vi "Config.vi"(8 "error in (no error)":errorcluster, 9 "Read only?":bool, 11 "STEP in":T1) -> (0 "error out":errorcluster, 1 "Discard?":bool=TRUE, 3 "STEP out":T1)   [LabVIEW 2014, in "SeqLoop.lvlib"]
uses:
  SeqLoop.lvlib
  TypeDefs/STEP.ctl
  TypeDefs/LogicParsedExpression.ctl
  Mimico Display/TypeDefs/Mimic Data.ctl
  Mimico Display/TypeDefs/BG Image.ctl
  Mimico Display/TypeDefs/mObject.ctl
  <vilib>/Utility/miscctls.llb/LVPointTypeDef.ctl
  Mimico Display/Mimico Display.lvlib
panel:
  in  "Reset?":bool
  in  "Number of STEPs":u32 caption="Cantidad de Pasos:"
  in  "Jump?":bool caption="Salto de Paso?"
  in  "Repetition":u32 caption="Nro. Repeticiones:"
  in  "Initial STEP":u32 caption="Punto de Salto:"
  out "Mimic Picture":picture
  in  "Mensaje de Error":string
  in  "Add Mimic":bool
  in  "Alarm Msj 4":string
  in  "Alarm Msj 3":string
  in  "Alarm Msj 2":string
  in  "Alarm Msj 1":string
  in  "Alarm 4":string
  in  "Alarm 3":string
  in  "Alarm 2":string
  in  "Alarm 1":string
  out "Paso:":u32
  in  "Mensaje al Operador":string
  in  "Condición de Error":string
  in  "S8:":i32
  in  "S7:":i32
  in  "S6:":i32
  in  "S5:":i32
  in  "S4:":i32
  in  "S3:":i32
  in  "S2:":i32
  in  "S1:":i32
  in  "Condición de Avance de Secuencia":string
  in  "Stop Med":bool
  in  "Add Med":bool
  # "Salto de Paso o Reset"
  # "Salidas Activadas"
  # "Gráfico Mimico"
  # "Alarma"
  # "Mensaje de Alarma"
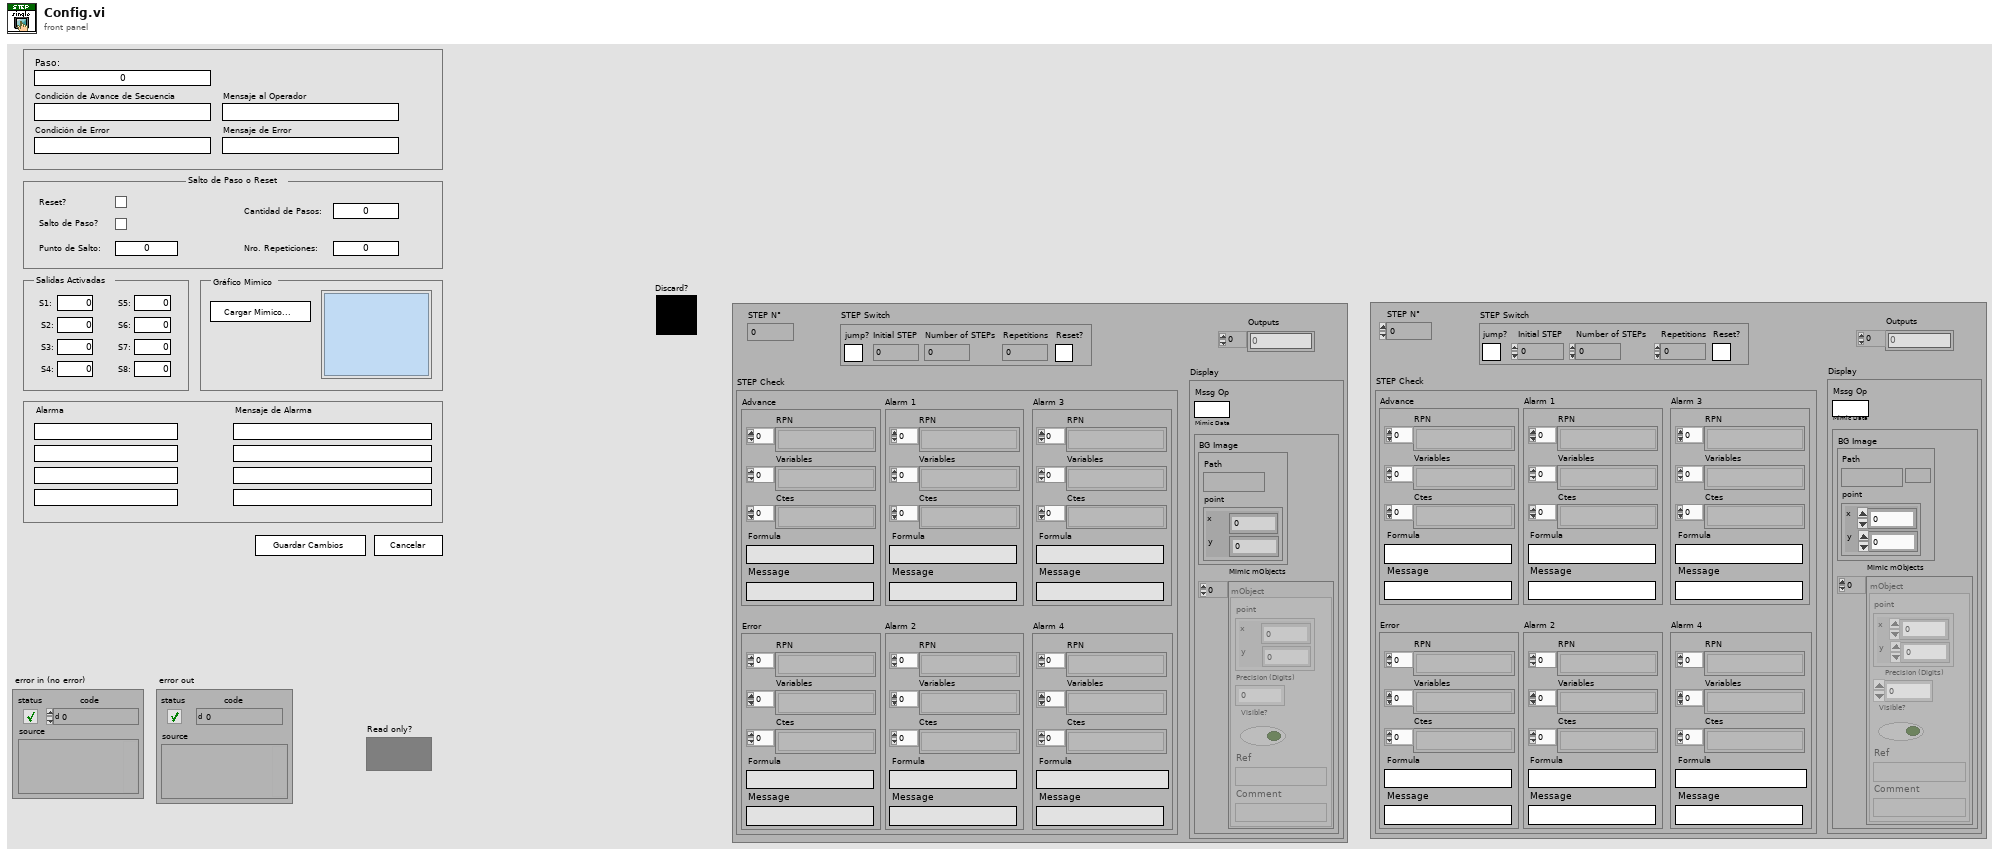
[diagram p1: front panel]
types:
  T1 = typedef "SeqLoop.lvlib/STEP.ctl" = cluster{"STEP N°":u32, "STEP Switch":cluster{"jump?":bool, "Initial STEP":u32, "Number of STEPs":u32, "Repetitions":u32, "Reset?":bool}, "Outputs":i32[], "STEP Check":cluster{"Advance":T2, "Error ":T2, "Alarm 1":T2, "Alarm 2":T2, "Alarm 3":T2, "Alarm 4":T2}, "Display":cluster{"Mssg Op":string, "Mimic Data":T3}}
  T2 = typedef "SeqLoop.lvlib/LogicParsedExpression.ctl" = cluster{"RPN ":string[], "Variables":string[], "Ctes":string[], "Formula":string, "Message":string}
  T3 = typedef "SeqLoop.lvlib/Mimico Display.lvlib/Mimic Data.ctl" = cluster{"BG Image":T4, "Mimic mObjects":T5[]}
  T4 = typedef "SeqLoop.lvlib/Mimico Display.lvlib/BG Image.ctl" = cluster{"Path":path, "point":cluster{"x":i16, "y":i16}}
  T5 = typedef "SeqLoop.lvlib/Mimico Display.lvlib/mObject.ctl" = cluster{"point":cluster{"x":i16, "y":i16}, "Precision (Digits)":i32, "Visible?":bool, "Ref":string, "Comment":string}
  T6 = typedef "LVPointTypeDef.ctl" = cluster{"Horizontal":i16, "Vertical":i16}
  T7 = enum8{"Enabled", "Disabled", "Disabled and Grayed Out"}
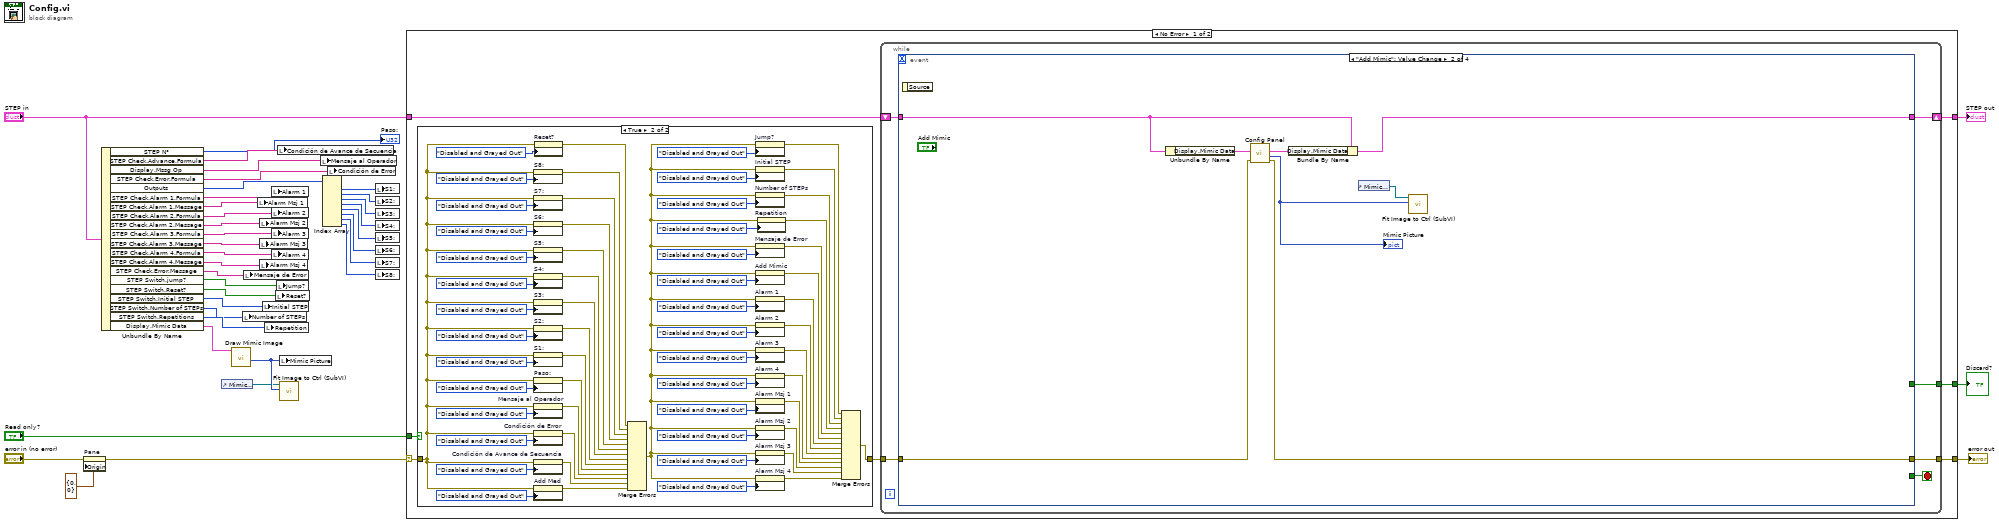
[diagram p0: block diagram]
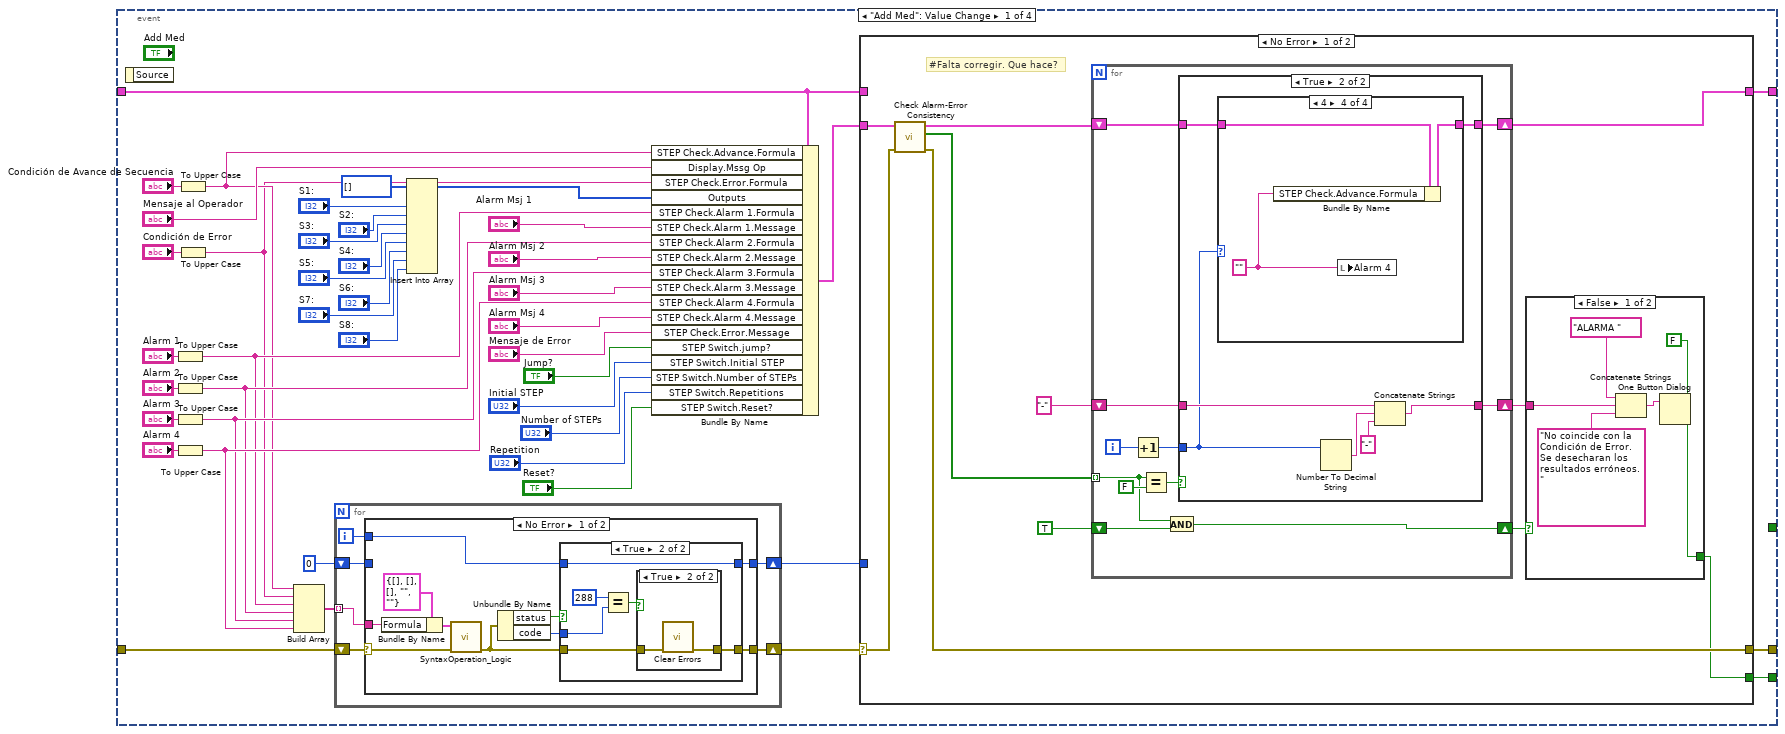
[diagram p3: hidden frame]
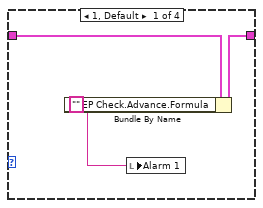
[diagram p5: hidden frame]
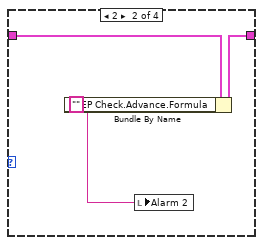
[diagram p6: hidden frame]
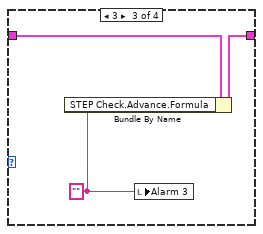
[diagram p7: hidden frame]
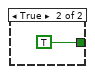
[diagram p8: hidden frame]
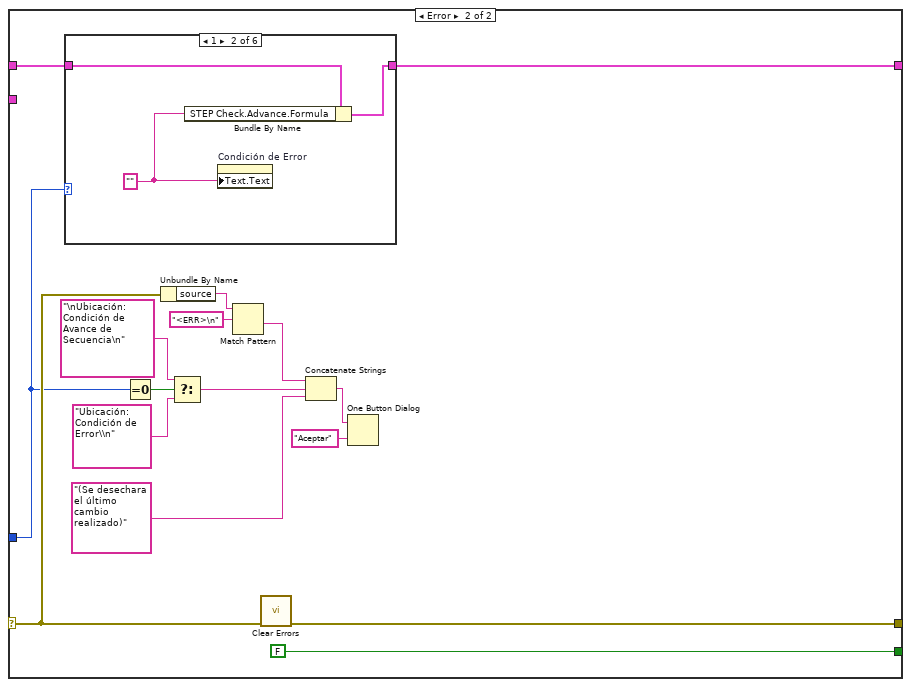
[diagram p9: hidden frame]
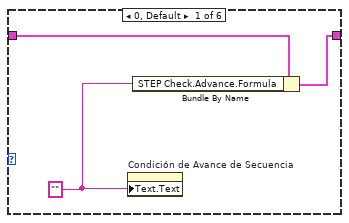
[diagram p10: hidden frame]
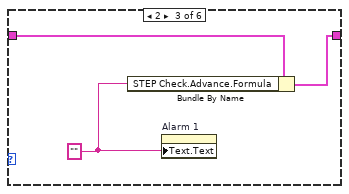
[diagram p11: hidden frame]
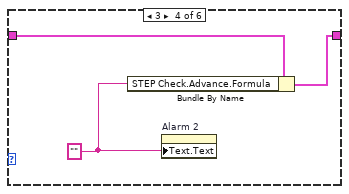
[diagram p12: hidden frame]
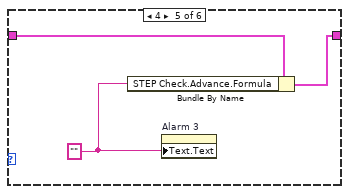
[diagram p13: hidden frame]
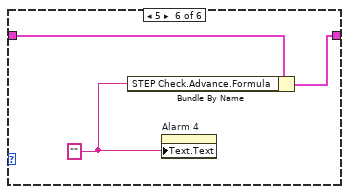
[diagram p14: hidden frame]
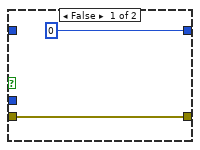
[diagram p15: hidden frame]
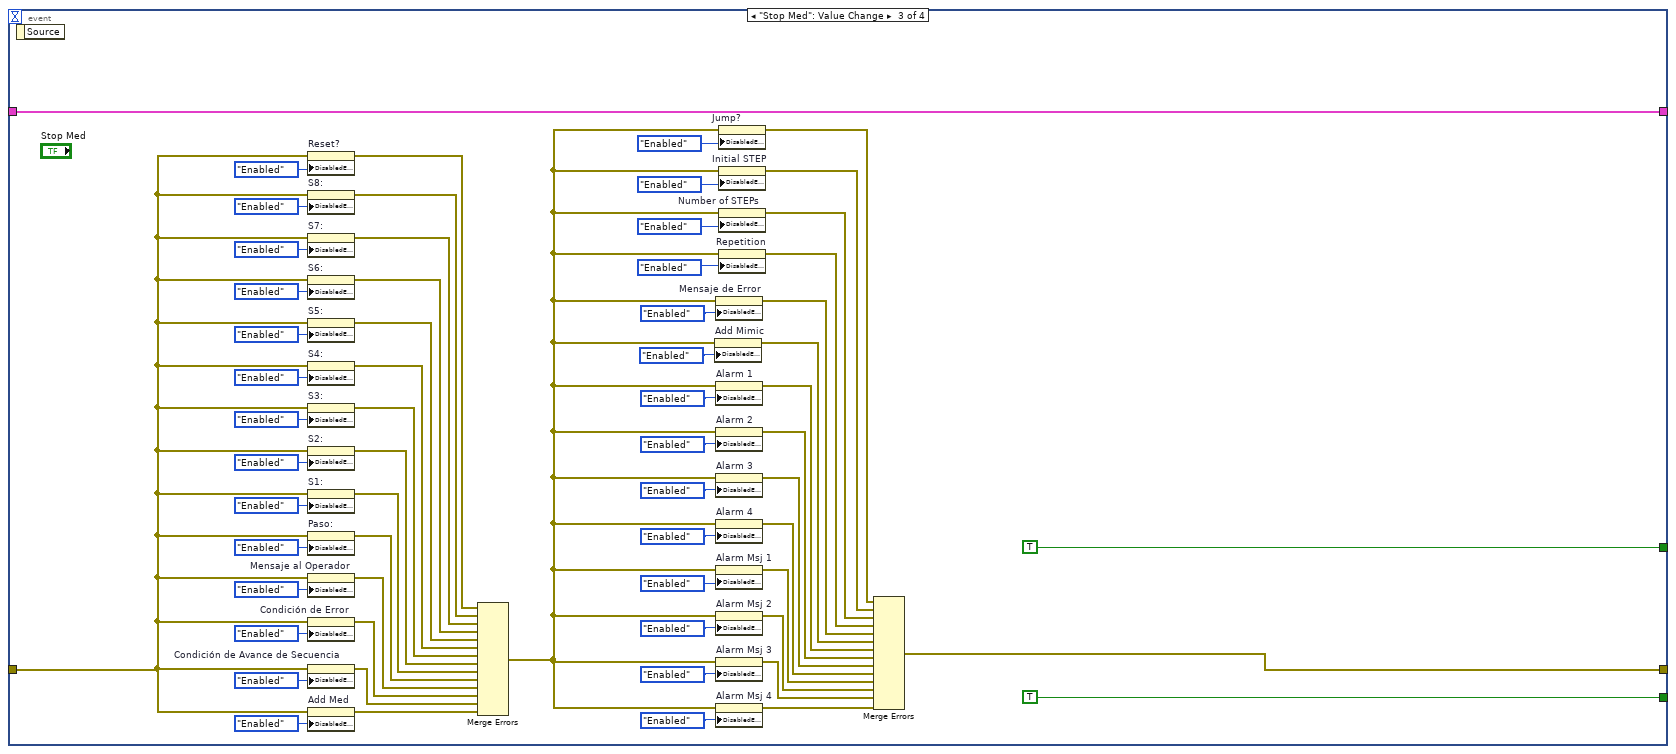
[diagram p18: hidden frame]
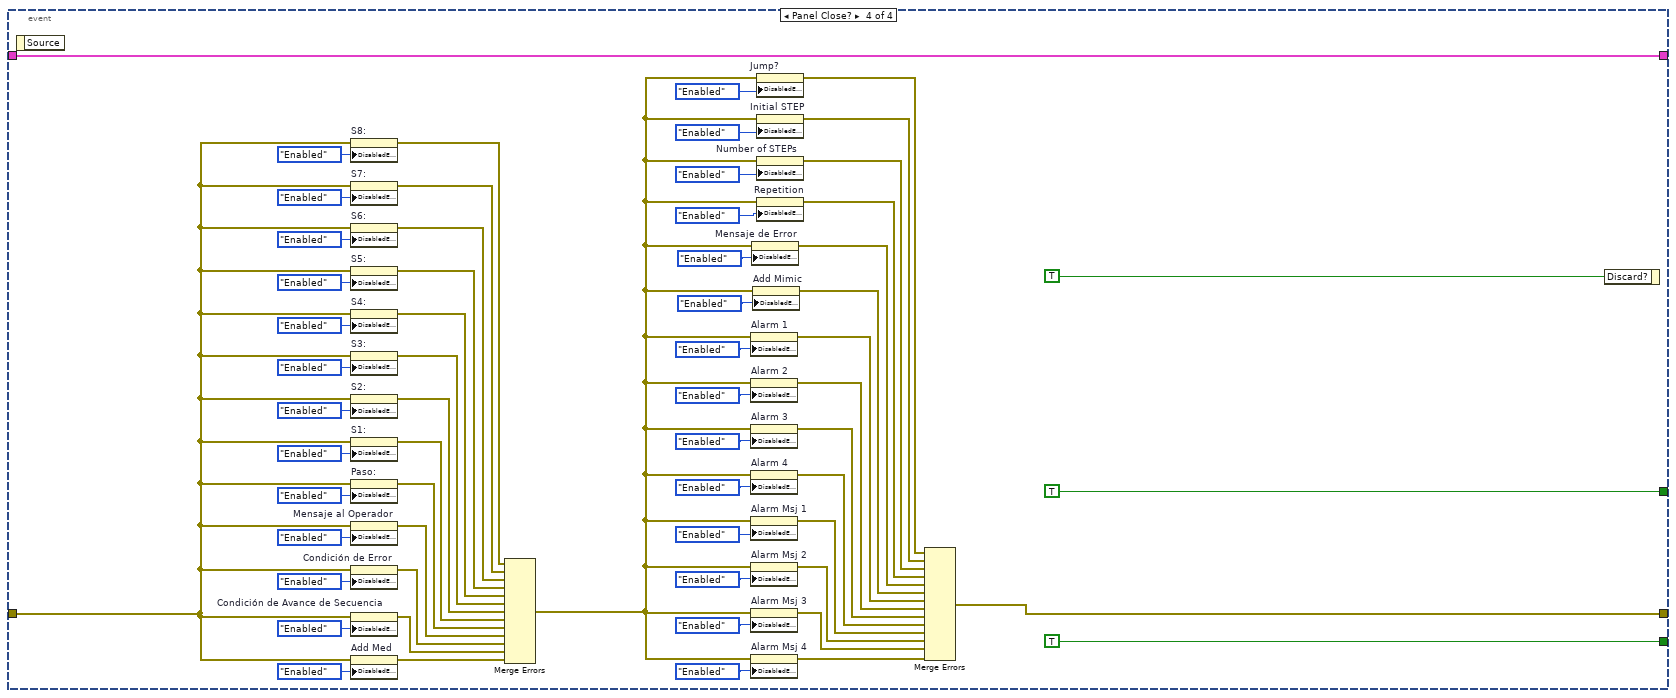
[diagram p19: hidden frame]
diagram:
  n1 = property on="Pane" class="Pane"(error in="error in (no error)", "Origin"=T6 {"Horizontal"=0, "Vertical"=0}) -> (error out=w11:errorcluster)  [unwired: 1 in, 1 out]
  n2 = Unbundle By Name("STEP in") -> ("STEP N°"=→"Paso:":u32, "STEP Check.Advance.Formula"=w36:string, "Display.Mssg Op"=w35:string, "STEP Check.Error.Formula"=w34:string, "Outputs"=w32:i32[], "STEP Check.Alarm 1.Formula"=w24:string, "STEP Check.Alarm 1.Message"=w23:string, "STEP Check.Alarm 2.Formula"=w22:string, "STEP Check.Alarm 2.Message"=w21:string, "STEP Check.Alarm 3.Formula"=w20:string, "STEP Check.Alarm 3.Message"=w17:string, "STEP Check.Alarm 4.Formula"=w18:string, "STEP Check.Alarm 4.Message"=w19:string, "STEP Check.Error.Message"=w16:string, "STEP Switch.jump?"=w10:bool, "STEP Switch.Reset?"=w4:bool, "STEP Switch.Initial STEP"=w5:u32, "STEP Switch.Number of STEPs"=w6:u32, "STEP Switch.Repetitions"=w7:u32, "Display.Mimic Data"=w8:T3)
  n3 = control-ref of="Mimic Picture"() -> (w14:refnum<vi>)
  n4 = call "Draw Mimic Image.vi"("Mimic Data in"=w8) -> ("Mimic Picture"=w15:picture)  [unwired: 10 in]
  n5 = local write "Number of STEPs"(w6) -> ()
  n6 = local write "Mensaje de Error"(w16) -> ()
  n7 = local write "Alarm Msj 1"(w23) -> ()
  n8 = local write "Alarm Msj 2"(w21) -> ()
  n9 = local write "Alarm Msj 3"(w17) -> ()
  n10 = local write "Alarm Msj 4"(w19) -> ()
  n11 = local write "Initial STEP"(w5) -> ()
  n12 = local write "Repetition"(w7) -> ()
  n13 = local write "Alarm 1"(w24) -> ()
  n14 = local write "Alarm 2"(w22) -> ()
  n15 = local write "Alarm 3"(w20) -> ()
  n16 = local write "Alarm 4"(w18) -> ()
  n17 = local write "Reset?"(w4) -> ()
  n18 = local write "Jump?"(w10) -> ()
  n19 = local write "Condición de Avance de Secuencia"(w36) -> ()
  n20 = call "Fit Image to Ctrl (SubVI).vi"("picture in"=w15, "Picture ref in"=w14) -> ()  [unwired: 10 in]
  n21 = local write "Mimic Picture"(w15) -> ()
  n22 = local write "Mensaje al Operador"(w35) -> ()
  n23 = Index Array(array=w32) -> (element #1=w33:i32, element #2=w31:i32, element #3=w30:i32, element #4=w29:i32, element #5=w28:i32, element #6=w27:i32, element #7=w26:i32, element #8=w25:i32)  [unwired: 8 in]
  n24 = local write "Condición de Error"(w34) -> ()
  n25 = local write "S1:"(w33) -> ()
  n26 = local write "S2:"(w31) -> ()
  n27 = local write "S3:"(w30) -> ()
  n28 = local write "S4:"(w29) -> ()
  n29 = local write "S5:"(w28) -> ()
  n30 = local write "S6:"(w27) -> ()
  n31 = local write "S7:"(w26) -> ()
  n32 = local write "S8:"(w25) -> ()
  n33 = case shown="No Error" w11 {
    selector: w11 -> [w43 w399]
    tunnel: [w45 w399] -> w38
    tunnel: "STEP in" -> [w40 w398]
    tunnel: [w44 w398] -> w1
    tunnel: "Read only?" -> [w41 _]
    tunnel: [w39 _] -> w9
    frame No Error {
      n34 = case shown="True" w41 {
        tunnel: w43 -> [w46 w48]
        tunnel: [w46 w79] -> w42
        frame False {
        }
        frame True {
          n35 = property on="S8:" class="DigNum (strict)"(error in=w48, "DisabledEnum"=T7."Disabled and Grayed Out" ("Disabled")) -> (error out=w83:errorcluster)  [unwired: 1 in, 1 out]
          n36 = property on="S7:" class="DigNum (strict)"(error in=w48, "DisabledEnum"=T7."Disabled and Grayed Out" ("Disabled")) -> (error out=w84:errorcluster)  [unwired: 1 in, 1 out]
          n37 = property on="S6:" class="DigNum (strict)"(error in=w48, "DisabledEnum"=T7."Disabled and Grayed Out" ("Disabled")) -> (error out=w85:errorcluster)  [unwired: 1 in, 1 out]
          n38 = property on="S5:" class="DigNum (strict)"(error in=w48, "DisabledEnum"=T7."Disabled and Grayed Out" ("Disabled")) -> (error out=w89:errorcluster)  [unwired: 1 in, 1 out]
          n39 = property on="S4:" class="DigNum (strict)"(error in=w48, "DisabledEnum"=T7."Disabled and Grayed Out" ("Disabled")) -> (error out=w90:errorcluster)  [unwired: 1 in, 1 out]
          n40 = property on="S3:" class="DigNum (strict)"(error in=w48, "DisabledEnum"=T7."Disabled and Grayed Out" ("Disabled")) -> (error out=w91:errorcluster)  [unwired: 1 in, 1 out]
          n41 = property on="S2:" class="DigNum (strict)"(error in=w48, "DisabledEnum"=T7."Disabled and Grayed Out" ("Disabled")) -> (error out=w92:errorcluster)  [unwired: 1 in, 1 out]
          n42 = property on="S1:" class="DigNum (strict)"(error in=w48, "DisabledEnum"=T7."Disabled and Grayed Out" ("Disabled")) -> (error out=w93:errorcluster)  [unwired: 1 in, 1 out]
          n43 = property on="Paso:" class="DigNum (strict)"(error in=w48, "DisabledEnum"=T7."Disabled and Grayed Out" ("Disabled")) -> (error out=w94:errorcluster)  [unwired: 1 in, 1 out]
          n44 = property on="Mensaje al Operador" class="Str"(error in=w48, "DisabledEnum"=T7."Disabled and Grayed Out" ("Disabled")) -> (error out=w95:errorcluster)  [unwired: 1 in, 1 out]
          n45 = property on="Condición de Error" class="Str"(error in=w48, "DisabledEnum"=T7."Disabled and Grayed Out" ("Disabled")) -> (error out=w88:errorcluster)  [unwired: 1 in, 1 out]
          n46 = property on="Condición de Avance de Secuencia" class="Str"(error in=w48, "DisabledEnum"=T7."Disabled and Grayed Out" ("Disabled")) -> (error out=w87:errorcluster)  [unwired: 1 in, 1 out]
          n47 = property on="Add Med" class="Bool"(error in=w48, "DisabledEnum"=T7."Disabled and Grayed Out" ("Disabled")) -> (error out=w86:errorcluster)  [unwired: 1 in, 1 out]
          n48 = property on="Reset?" class="Bool (strict)"(error in=w48, "DisabledEnum"=T7."Disabled and Grayed Out" ("Disabled")) -> (error out=w47:errorcluster)  [unwired: 1 in, 1 out]
          n49 = Merge Errors(w47, w83, w84, w85, w89, w90, w91, w92, w93, w94, w95, w88, w87, w86) -> (w51:errorcluster)
          n50 = property on="Jump?" class="Bool (strict)"(error in=w51, "DisabledEnum"=T7."Disabled and Grayed Out" ("Disabled")) -> (error out=w50:errorcluster)  [unwired: 1 in, 1 out]
          n51 = property on="Initial STEP" class="DigNum (strict)"(error in=w51, "DisabledEnum"=T7."Disabled and Grayed Out" ("Disabled")) -> (error out=w53:errorcluster)  [unwired: 1 in, 1 out]
          n52 = property on="Number of STEPs" class="DigNum (strict)"(error in=w51, "DisabledEnum"=T7."Disabled and Grayed Out" ("Disabled")) -> (error out=w54:errorcluster)  [unwired: 1 in, 1 out]
          n53 = property on="Mensaje de Error" class="Str"(error in=w51, "DisabledEnum"=T7."Disabled and Grayed Out" ("Disabled")) -> (error out=w59:errorcluster)  [unwired: 1 in, 1 out]
          n54 = property on="Add Mimic" class="Bool"(error in=w51, "DisabledEnum"=T7."Disabled and Grayed Out" ("Disabled")) -> (error out=w62:errorcluster)  [unwired: 1 in, 1 out]
          n55 = property on="Alarm 1" class="Str"(error in=w51, "DisabledEnum"=T7."Disabled and Grayed Out" ("Disabled")) -> (error out=w71:errorcluster)  [unwired: 1 in, 1 out]
          n56 = property on="Alarm 2" class="Str"(error in=w51, "DisabledEnum"=T7."Disabled and Grayed Out" ("Disabled")) -> (error out=w72:errorcluster)  [unwired: 1 in, 1 out]
          n57 = property on="Alarm 3" class="Str"(error in=w51, "DisabledEnum"=T7."Disabled and Grayed Out" ("Disabled")) -> (error out=w73:errorcluster)  [unwired: 1 in, 1 out]
          n58 = property on="Alarm 4" class="Str"(error in=w51, "DisabledEnum"=T7."Disabled and Grayed Out" ("Disabled")) -> (error out=w74:errorcluster)  [unwired: 1 in, 1 out]
          n59 = property on="Alarm Msj 1" class="Str"(error in=w51, "DisabledEnum"=T7."Disabled and Grayed Out" ("Disabled")) -> (error out=w75:errorcluster)  [unwired: 1 in, 1 out]
          n60 = property on="Alarm Msj 2" class="Str"(error in=w51, "DisabledEnum"=T7."Disabled and Grayed Out" ("Disabled")) -> (error out=w76:errorcluster)  [unwired: 1 in, 1 out]
          n61 = property on="Alarm Msj 3" class="Str"(error in=w51, "DisabledEnum"=T7."Disabled and Grayed Out" ("Disabled")) -> (error out=w77:errorcluster)  [unwired: 1 in, 1 out]
          n62 = property on="Alarm Msj 4" class="Str"(error in=w51, "DisabledEnum"=T7."Disabled and Grayed Out" ("Disabled")) -> (error out=w78:errorcluster)  [unwired: 1 in, 1 out]
          n63 = property on="Repetition" class="DigNum (strict)"(error in=w51, "DisabledEnum"=T7."Disabled and Grayed Out" ("Disabled")) -> (error out=w55:errorcluster)  [unwired: 1 in, 1 out]
          n64 = Merge Errors(w50, w53, w54, w55, w59, w62, w71, w72, w73, w74, w75, w76, w77, w78) -> (w79:errorcluster)
        }
      }
      n65 = while {
        tunnel: w42 -> [w110]
        tunnel: [w111] -> w45
        shift-right: [w107] -> w44
        shift-left: w40 -> [w108]
        tunnel: [w106] -> w39
        stop <- w109 stop-if-true
        n66 = event shown="[1] \"Add Mimic\": Value Change" {
          selector: _ -> [_ _ _ _]
          dyn-events: _ -> [_ _ _ _]
          timeout: _ -> [_ _ _ _]
          tunnel: [w139 w272 w293 w351] -> w111
          tunnel: w110 -> [w137 w273 w276 w352]
          tunnel: [w136 _ TRUE ("Discard?") TRUE ("Discard?")] -> w109
          tunnel: w108 -> [w140 w271 w279 w395]
          tunnel: [w141 w269 w279 w395] -> w107
          tunnel: [_ _ TRUE ("Discard? 2") TRUE ("Discard? 2")] -> w106
          event "Add Med": Value Change {
            n67 = event-data() -> ()  [unwired: 1 in, 1 out]
            n68 = To Upper Case(1:"Alarm 1") -> (0:w115:string)
            n69 = To Upper Case(1:"Alarm 2") -> (0:w116:string)
            n70 = To Upper Case(1:"Alarm 3") -> (0:w117:string)
            n71 = To Upper Case(1:"Alarm 4") -> (0:w118:string)
            n72 = To Upper Case(1:"Condición de Avance de Secuencia") -> (0:w114:string)
            n73 = To Upper Case(1:"Condición de Error") -> (0:w113:string)
            n74 = Build Array(w114, w113, w115, w116, w117, w118) -> (w143:string[])
            n75 = for {
              tunnel: w143 -> [w243] mode=indexing
              shift-right: [w242] -> w138
              shift-left: w137 -> [w240]
              shift-right: [w239] -> w134
              shift-left: 0 -> [w238]
              i -> [w241]
              n76 = case shown="No Error" w240 {
                selector: w240 -> [w246 w266]
                tunnel: w243 -> [w251 _]
                tunnel: [w249 w266] -> w242
                tunnel: w241 -> [w247 _]
                tunnel: [w245 w265] -> w239
                tunnel: w238 -> [_ w265]
                frame No Error {
                  n77 = Bundle By Name(cluster=T2 {"RPN "=[], "Variables"=[], "Ctes"=[], "Formula"="", "Message"=""} ("Logical Parsed Expression"), "Formula"=w251) -> (w252:T2)
                  n78 = call "SyntaxOperation_Logic.vi"("error in (no error)"=w246, "Logical Parsed Expression"=w252) -> ("error out"=w248:errorcluster)  [unwired: 6 in, 3 out]
                  n79 = Unbundle By Name(w248) -> ("status"=w250:bool, "code"=w244:i32)
                  n80 = case shown="True" w250 {
                    tunnel: [w255 w256] -> w249
                    tunnel: w248 -> [w255 w257]
                    tunnel: w247 -> [_ w261]
                    tunnel: [0 w261] -> w245
                    tunnel: w244 -> [_ w260]
                    frame False {
                    }
                    frame True {
                      n81 = Equal?(x=288, y=w260) -> (x = y?=w258:bool)
                      n82 = case shown="True" w258 {
                        tunnel: w257 -> [w262 w264]
                        tunnel: [w262 w263] -> w256
                        frame False {
                        }
                        frame True {
                          n83 = call <vilib>:"Clear Errors.vi"("error in (no error)"=w264) -> ("error out"=w263:errorcluster)  [unwired: 5 in, 1 out]
                        }
                      }
                    }
                  }
                }
                frame Error {
                }
              }
            }
            n84 = Insert Into Array(array=i32[] [] ("Outputs"), new element #1="S1:", new element #2="S2:", new element #3="S3:", new element #4="S4:", new element #5="S5:", new element #6="S6:", new element #7="S7:", new element #8="S8:") -> (w144:i32[])  [unwired: 1 in]
            n85 = Bundle By Name(cluster=w140, "STEP Check.Advance.Formula"=w114, "Display.Mssg Op"="Mensaje al Operador", "STEP Check.Error.Formula"=w113, "Outputs"=w144, "STEP Check.Alarm 1.Formula"=w115, "STEP Check.Alarm 1.Message"="Alarm Msj 1", "STEP Check.Alarm 2.Formula"=w116, "STEP Check.Alarm 2.Message"="Alarm Msj 2", "STEP Check.Alarm 3.Formula"=w117, "STEP Check.Alarm 3.Message"="Alarm Msj 3", "STEP Check.Alarm 4.Formula"=w118, "STEP Check.Alarm 4.Message"="Alarm Msj 4", "STEP Check.Error.Message"="Mensaje de Error", "STEP Switch.jump?"="Jump?", "STEP Switch.Initial STEP"="Initial STEP", "STEP Switch.Number of STEPs"="Number of STEPs", "STEP Switch.Repetitions"="Repetition", "STEP Switch.Reset?"="Reset?") -> (w142:T1)
            n86 = case shown="No Error" w138 {
              selector: w138 -> [w160 w214]
              tunnel: w142 -> [w158 _]
              tunnel: [w161 w210] -> w141
              tunnel: w140 -> [_ w211]
              tunnel: [w159 w213] -> w139
              tunnel: [w155 FALSE ("Discard?")] -> w136
              tunnel: w134 -> [_ w207]
              frame No Error {
                # "#Falta corregir. Que hace?"
                n87 = call "Check Alarm-Error Consistency.vi"("error in (no error)"=w160, "STEP In"=w158) -> ("error out"=w159:errorcluster, "Array"=w156:bool[], "STEP out"=w157:T1)  [unwired: 7 in]
                n88 = for {
                  tunnel: w156 -> [w168] mode=indexing
                  shift-right: [w176] -> w164
                  shift-left: TRUE -> [w169]
                  shift-right: [w170] -> w162
                  shift-left: "-" ("string") -> [w171]
                  shift-right: [w167] -> w161
                  shift-left: w157 -> [w166]
                  i -> [w173]
                  n89 = Increment(x=w173) -> (x+1=w172:i32)
                  n90 = Equal?(x=w168, y=FALSE) -> (x = y?=w174:bool)
                  n91 = And(x=w168, y=w169) -> (x .and. y?=w176:bool)
                  n92 = case shown="True" w174 {
                    tunnel: w172 -> [_ w181]
                    tunnel: w171 -> [w178 w184]
                    tunnel: [w178 w183] -> w170
                    tunnel: [w177 w180] -> w167
                    tunnel: w166 -> [w177 w179]
                    frame False {
                    }
                    frame True {
                      n93 = case shown="4" w181 {
                        tunnel: [w188 w191 w194 w197] -> w180
                        tunnel: w179 -> [w187 w190 w193 w196]
                        frame 1, Default {
                          w186 = "" ("Alarm 1.Formula")
                          n94 = Bundle By Name(cluster=w187, "STEP Check.Advance.Formula"=w186) -> (w188:T1)
                          n95 = local write "Alarm 1"(w186) -> ()
                        }
                        frame 2 {
                          w189 = "" ("Alarm 1.Formula")
                          n96 = Bundle By Name(cluster=w190, "STEP Check.Advance.Formula"=w189) -> (w191:T1)
                          n97 = local write "Alarm 2"(w189) -> ()
                        }
                        frame 3 {
                          w192 = "" ("Alarm 1.Formula")
                          n98 = Bundle By Name(cluster=w193, "STEP Check.Advance.Formula"=w192) -> (w194:T1)
                          n99 = local write "Alarm 3"(w192) -> ()
                        }
                        frame 4 {
                          w195 = "" ("Alarm 1.Formula")
                          n100 = Bundle By Name(cluster=w196, "STEP Check.Advance.Formula"=w195) -> (w197:T1)
                          n101 = local write "Alarm 4"(w195) -> ()
                        }
                      }
                      n102 = Number To Decimal String(number=w181) -> (decimal integer string=w185:string)  [unwired: 1 in]
                      n103 = Concatenate Strings(w184, w185, "-" ("string")) -> (w183:string)
                    }
                  }
                }
                n104 = case shown="False" w164 {
                  tunnel: [FALSE TRUE] -> w155
                  tunnel: w162 -> [w200 _]
                  frame False {
                    n105 = Concatenate Strings("ALARMA " ("message"), w200, "No coincide con la Condición de Error. Se desecharan los resultados erróneos." ("string")) -> (w199:string)
                    n106 = One Button Dialog(message=w199) -> ()  [unwired: 1 in, 1 out]
                  }
                  frame True {
                  }
                }
              }
              frame Error {
                n107 = case shown="1" w207 {
                  tunnel: w211 -> [w222 w225 w228 w231 w234 w237]
                  tunnel: [w221 w224 w227 w230 w233 w236] -> w210
                  frame 0, Default {
                    w220 = "" ("Text.Text")
                    n108 = property on="Condición de Avance de Secuencia" class="Str"("Text.Text"=w220) -> ()  [unwired: 2 in, 2 out]
                    n109 = Bundle By Name(cluster=w222, "STEP Check.Advance.Formula"=w220) -> (w221:T1)
                  }
                  frame 1 {
                    w223 = "" ("Text.Text")
                    n110 = Bundle By Name(cluster=w225, "STEP Check.Advance.Formula"=w223) -> (w224:T1)
                    n111 = property on="Condición de Error" class="Str"("Text.Text"=w223) -> ()  [unwired: 2 in, 2 out]
                  }
                  frame 2 {
                    w226 = "" ("Text.Text")
                    n112 = Bundle By Name(cluster=w228, "STEP Check.Advance.Formula"=w226) -> (w227:T1)
                    n113 = property on="Alarm 1" class="Str"("Text.Text"=w226) -> ()  [unwired: 2 in, 2 out]
                  }
                  frame 3 {
                    w229 = "" ("Text.Text")
                    n114 = Bundle By Name(cluster=w231, "STEP Check.Advance.Formula"=w229) -> (w230:T1)
                    n115 = property on="Alarm 2" class="Str"("Text.Text"=w229) -> ()  [unwired: 2 in, 2 out]
                  }
                  frame 4 {
                    w232 = "" ("Text.Text")
                    n116 = Bundle By Name(cluster=w234, "STEP Check.Advance.Formula"=w232) -> (w233:T1)
                    n117 = property on="Alarm 3" class="Str"("Text.Text"=w232) -> ()  [unwired: 2 in, 2 out]
                  }
                  frame 5 {
                    w235 = "" ("Text.Text")
                    n118 = Bundle By Name(cluster=w237, "STEP Check.Advance.Formula"=w235) -> (w236:T1)
                    n119 = property on="Alarm 4" class="Str"("Text.Text"=w235) -> ()  [unwired: 2 in, 2 out]
                  }
                }
                n120 = Equal To 0?(x=w207) -> (x = 0?=w208:bool)
                n121 = Unbundle By Name(w214) -> ("source"=w216:string)
                n122 = Select(t="\nUbicación: Condición de Avance de Secuencia\n" ("regular expression"), s=w208, f="Ubicación: Condición de Error\\n" ("regular expression")) -> (s? t:f=w206:string)
                n123 = Match Pattern(string=w216, regular expression="<ERR>\n") -> (after substring=w218:string)  [unwired: 1 in, 3 out]
                n124 = call <vilib>:"Clear Errors.vi"("error in (no error)"=w214) -> ("error out"=w213:errorcluster)  [unwired: 5 in, 1 out]
                n125 = Concatenate Strings(w218, w206, "(Se desechara el último cambio realizado)" ("button name (\"OK\")")) -> (w219:string)
                n126 = One Button Dialog(message=w219, button name ("OK")="Aceptar") -> ()  [unwired: 1 out]
              }
            }
          }
          event "Add Mimic": Value Change {
            n127 = event-data() -> ()  [unwired: 1 in, 1 out]
            n128 = Unbundle By Name(w271) -> ("Display.Mimic Data"=w274:T3)
            n129 = call "Config Panel.vi"("error in (no error)"=w273, "Mimic Data in"=w274) -> ("error out"=w272:errorcluster, "Mimic Picture"=w268:picture, "Mimic Data out"=w270:T3)  [unwired: 7 in]
            "Mimic Picture" <- w268
            n130 = Bundle By Name(cluster=w271, "Display.Mimic Data"=w270) -> (w269:T1)
            n131 = control-ref of="Mimic Picture"() -> (w267:refnum<vi>)
            n132 = call "Fit Image to Ctrl (SubVI).vi"("picture in"=w268, "Picture ref in"=w267) -> ()  [unwired: 10 in]
          }
          event "Stop Med": Value Change {
            n133 = event-data() -> ()  [unwired: 1 in, 1 out]
            n134 = property on="Reset?" class="Bool (strict)"(error in=w276, "DisabledEnum"=T7."Enabled" ("Disabled")) -> (error out=w275:errorcluster)  [unwired: 1 in, 1 out]
            n135 = property on="S8:" class="DigNum (strict)"(error in=w276, "DisabledEnum"=T7."Enabled" ("Disabled")) -> (error out=w316:errorcluster)  [unwired: 1 in, 1 out]
            n136 = property on="S7:" class="DigNum (strict)"(error in=w276, "DisabledEnum"=T7."Enabled" ("Disabled")) -> (error out=w315:errorcluster)  [unwired: 1 in, 1 out]
            n137 = property on="S6:" class="DigNum (strict)"(error in=w276, "DisabledEnum"=T7."Enabled" ("Disabled")) -> (error out=w314:errorcluster)  [unwired: 1 in, 1 out]
            n138 = property on="S5:" class="DigNum (strict)"(error in=w276, "DisabledEnum"=T7."Enabled" ("Disabled")) -> (error out=w310:errorcluster)  [unwired: 1 in, 1 out]
            n139 = property on="S4:" class="DigNum (strict)"(error in=w276, "DisabledEnum"=T7."Enabled" ("Disabled")) -> (error out=w309:errorcluster)  [unwired: 1 in, 1 out]
            n140 = property on="S3:" class="DigNum (strict)"(error in=w276, "DisabledEnum"=T7."Enabled" ("Disabled")) -> (error out=w308:errorcluster)  [unwired: 1 in, 1 out]
            n141 = property on="S2:" class="DigNum (strict)"(error in=w276, "DisabledEnum"=T7."Enabled" ("Disabled")) -> (error out=w307:errorcluster)  [unwired: 1 in, 1 out]
            n142 = property on="S1:" class="DigNum (strict)"(error in=w276, "DisabledEnum"=T7."Enabled" ("Disabled")) -> (error out=w306:errorcluster)  [unwired: 1 in, 1 out]
            n143 = property on="Paso:" class="DigNum (strict)"(error in=w276, "DisabledEnum"=T7."Enabled" ("Disabled")) -> (error out=w305:errorcluster)  [unwired: 1 in, 1 out]
            n144 = property on="Mensaje al Operador" class="Str"(error in=w276, "DisabledEnum"=T7."Enabled" ("Disabled")) -> (error out=w304:errorcluster)  [unwired: 1 in, 1 out]
            n145 = property on="Condición de Error" class="Str"(error in=w276, "DisabledEnum"=T7."Enabled" ("Disabled")) -> (error out=w311:errorcluster)  [unwired: 1 in, 1 out]
            n146 = property on="Condición de Avance de Secuencia" class="Str"(error in=w276, "DisabledEnum"=T7."Enabled" ("Disabled")) -> (error out=w312:errorcluster)  [unwired: 1 in, 1 out]
            n147 = property on="Add Med" class="Bool"(error in=w276, "DisabledEnum"=T7."Enabled" ("Disabled")) -> (error out=w313:errorcluster)  [unwired: 1 in, 1 out]
            n148 = Merge Errors(w275, w316, w315, w314, w310, w309, w308, w307, w306, w305, w304, w311, w312, w313) -> (w281:errorcluster)
            n149 = property on="Add Mimic" class="Bool"(error in=w281, "DisabledEnum"=T7."Enabled" ("Disabled")) -> (error out=w291:errorcluster)  [unwired: 1 in, 1 out]
            n150 = property on="Mensaje de Error" class="Str"(error in=w281, "DisabledEnum"=T7."Enabled" ("Disabled")) -> (error out=w290:errorcluster)  [unwired: 1 in, 1 out]
            n151 = property on="Alarm 1" class="Str"(error in=w281, "DisabledEnum"=T7."Enabled" ("Disabled")) -> (error out=w327:errorcluster)  [unwired: 1 in, 1 out]
            n152 = property on="Alarm 2" class="Str"(error in=w281, "DisabledEnum"=T7."Enabled" ("Disabled")) -> (error out=w326:errorcluster)  [unwired: 1 in, 1 out]
            n153 = property on="Alarm 3" class="Str"(error in=w281, "DisabledEnum"=T7."Enabled" ("Disabled")) -> (error out=w325:errorcluster)  [unwired: 1 in, 1 out]
            n154 = property on="Alarm 4" class="Str"(error in=w281, "DisabledEnum"=T7."Enabled" ("Disabled")) -> (error out=w324:errorcluster)  [unwired: 1 in, 1 out]
            n155 = property on="Alarm Msj 1" class="Str"(error in=w281, "DisabledEnum"=T7."Enabled" ("Disabled")) -> (error out=w323:errorcluster)  [unwired: 1 in, 1 out]
            n156 = property on="Alarm Msj 2" class="Str"(error in=w281, "DisabledEnum"=T7."Enabled" ("Disabled")) -> (error out=w322:errorcluster)  [unwired: 1 in, 1 out]
            n157 = property on="Alarm Msj 3" class="Str"(error in=w281, "DisabledEnum"=T7."Enabled" ("Disabled")) -> (error out=w321:errorcluster)  [unwired: 1 in, 1 out]
            n158 = property on="Alarm Msj 4" class="Str"(error in=w281, "DisabledEnum"=T7."Enabled" ("Disabled")) -> (error out=w320:errorcluster)  [unwired: 1 in, 1 out]
            n159 = property on="Jump?" class="Bool (strict)"(error in=w281, "DisabledEnum"=T7."Enabled" ("Disabled")) -> (error out=w282:errorcluster)  [unwired: 1 in, 1 out]
            n160 = property on="Initial STEP" class="DigNum (strict)"(error in=w281, "DisabledEnum"=T7."Enabled" ("Disabled")) -> (error out=w283:errorcluster)  [unwired: 1 in, 1 out]
            n161 = property on="Number of STEPs" class="DigNum (strict)"(error in=w281, "DisabledEnum"=T7."Enabled" ("Disabled")) -> (error out=w284:errorcluster)  [unwired: 1 in, 1 out]
            n162 = property on="Repetition" class="DigNum (strict)"(error in=w281, "DisabledEnum"=T7."Enabled" ("Disabled")) -> (error out=w285:errorcluster)  [unwired: 1 in, 1 out]
            n163 = Merge Errors(w282, w283, w284, w285, w290, w291, w327, w326, w325, w324, w323, w322, w321, w320) -> (w293:errorcluster)
          }
          event Panel Close? {
            n164 = event-data() -> ()  [unwired: 1 in, 1 out]
            n165 = property on="S8:" class="DigNum (strict)"(error in=w352, "DisabledEnum"=T7."Enabled" ("Disabled")) -> (error out=w375:errorcluster)  [unwired: 1 in, 1 out]
            n166 = property on="S7:" class="DigNum (strict)"(error in=w352, "DisabledEnum"=T7."Enabled" ("Disabled")) -> (error out=w374:errorcluster)  [unwired: 1 in, 1 out]
            n167 = property on="S6:" class="DigNum (strict)"(error in=w352, "DisabledEnum"=T7."Enabled" ("Disabled")) -> (error out=w373:errorcluster)  [unwired: 1 in, 1 out]
            n168 = property on="S5:" class="DigNum (strict)"(error in=w352, "DisabledEnum"=T7."Enabled" ("Disabled")) -> (error out=w369:errorcluster)  [unwired: 1 in, 1 out]
            n169 = property on="S4:" class="DigNum (strict)"(error in=w352, "DisabledEnum"=T7."Enabled" ("Disabled")) -> (error out=w368:errorcluster)  [unwired: 1 in, 1 out]
            n170 = property on="S3:" class="DigNum (strict)"(error in=w352, "DisabledEnum"=T7."Enabled" ("Disabled")) -> (error out=w367:errorcluster)  [unwired: 1 in, 1 out]
            n171 = property on="S2:" class="DigNum (strict)"(error in=w352, "DisabledEnum"=T7."Enabled" ("Disabled")) -> (error out=w366:errorcluster)  [unwired: 1 in, 1 out]
            n172 = property on="S1:" class="DigNum (strict)"(error in=w352, "DisabledEnum"=T7."Enabled" ("Disabled")) -> (error out=w365:errorcluster)  [unwired: 1 in, 1 out]
            n173 = property on="Paso:" class="DigNum (strict)"(error in=w352, "DisabledEnum"=T7."Enabled" ("Disabled")) -> (error out=w364:errorcluster)  [unwired: 1 in, 1 out]
            n174 = property on="Mensaje al Operador" class="Str"(error in=w352, "DisabledEnum"=T7."Enabled" ("Disabled")) -> (error out=w363:errorcluster)  [unwired: 1 in, 1 out]
            n175 = property on="Condición de Error" class="Str"(error in=w352, "DisabledEnum"=T7."Enabled" ("Disabled")) -> (error out=w370:errorcluster)  [unwired: 1 in, 1 out]
            n176 = property on="Condición de Avance de Secuencia" class="Str"(error in=w352, "DisabledEnum"=T7."Enabled" ("Disabled")) -> (error out=w371:errorcluster)  [unwired: 1 in, 1 out]
            n177 = property on="Add Med" class="Bool"(error in=w352, "DisabledEnum"=T7."Enabled" ("Disabled")) -> (error out=w372:errorcluster)  [unwired: 1 in, 1 out]
            n178 = Merge Errors(w375, w374, w373, w369, w368, w367, w366, w365, w364, w363, w370, w371, w372) -> (w338:errorcluster)
            n179 = property on="Alarm 1" class="Str"(error in=w338, "DisabledEnum"=T7."Enabled" ("Disabled")) -> (error out=w386:errorcluster)  [unwired: 1 in, 1 out]
            n180 = property on="Alarm 2" class="Str"(error in=w338, "DisabledEnum"=T7."Enabled" ("Disabled")) -> (error out=w385:errorcluster)  [unwired: 1 in, 1 out]
            n181 = property on="Alarm 3" class="Str"(error in=w338, "DisabledEnum"=T7."Enabled" ("Disabled")) -> (error out=w384:errorcluster)  [unwired: 1 in, 1 out]
            n182 = property on="Alarm 4" class="Str"(error in=w338, "DisabledEnum"=T7."Enabled" ("Disabled")) -> (error out=w383:errorcluster)  [unwired: 1 in, 1 out]
            n183 = property on="Alarm Msj 1" class="Str"(error in=w338, "DisabledEnum"=T7."Enabled" ("Disabled")) -> (error out=w382:errorcluster)  [unwired: 1 in, 1 out]
            n184 = property on="Alarm Msj 2" class="Str"(error in=w338, "DisabledEnum"=T7."Enabled" ("Disabled")) -> (error out=w381:errorcluster)  [unwired: 1 in, 1 out]
            n185 = property on="Alarm Msj 3" class="Str"(error in=w338, "DisabledEnum"=T7."Enabled" ("Disabled")) -> (error out=w380:errorcluster)  [unwired: 1 in, 1 out]
            n186 = property on="Alarm Msj 4" class="Str"(error in=w338, "DisabledEnum"=T7."Enabled" ("Disabled")) -> (error out=w379:errorcluster)  [unwired: 1 in, 1 out]
            n187 = property on="Mensaje de Error" class="Str"(error in=w338, "DisabledEnum"=T7."Enabled" ("Disabled")) -> (error out=w347:errorcluster)  [unwired: 1 in, 1 out]
            n188 = property on="Add Mimic" class="Bool"(error in=w338, "DisabledEnum"=T7."Enabled" ("Disabled")) -> (error out=w349:errorcluster)  [unwired: 1 in, 1 out]
            n189 = property on="Jump?" class="Bool (strict)"(error in=w338, "DisabledEnum"=T7."Enabled" ("Disabled")) -> (error out=w339:errorcluster)  [unwired: 1 in, 1 out]
            n190 = property on="Initial STEP" class="DigNum (strict)"(error in=w338, "DisabledEnum"=T7."Enabled" ("Disabled")) -> (error out=w340:errorcluster)  [unwired: 1 in, 1 out]
            n191 = property on="Number of STEPs" class="DigNum (strict)"(error in=w338, "DisabledEnum"=T7."Enabled" ("Disabled")) -> (error out=w341:errorcluster)  [unwired: 1 in, 1 out]
            n192 = property on="Repetition" class="DigNum (strict)"(error in=w338, "DisabledEnum"=T7."Enabled" ("Disabled")) -> (error out=w342:errorcluster)  [unwired: 1 in, 1 out]
            n193 = Merge Errors(w339, w340, w341, w342, w347, w349, w386, w385, w384, w383, w382, w381, w380, w379) -> (w351:errorcluster)
            n194 = event-data("Discard?"=TRUE) -> ()  [unwired: 1 in, 1 out]
          }
        }
      }
    }
    frame Error {
    }
  }
  "error out" <- w38
  "Discard?" <- w9
  "STEP out" <- w1
